vi "Get Stock Prices.vi"(11 "time":i32) -> (3 "Prices":dbl[](array[numeric]))   [LabVIEW 2025, in "Full Featured MCP Server.lvlib"]
doc: "Teturns all prices of the stocks for a specific point in time. Use this twice to compare price changes."
uses:
  Full Featured MCP Server.lvlib
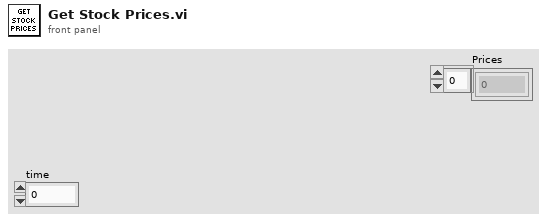
[diagram p1: front panel]
types:
  T1 = typedef "Full Featured MCP Server.lvlib/Server Data.ctl" = cluster{"Stocks Prices":dbl[][], "Owned Stocks":i32[], "Stock Names":string[], "Wallet":dbl, "Fluctuation":dbl, "Stock Trends":dbl[]}
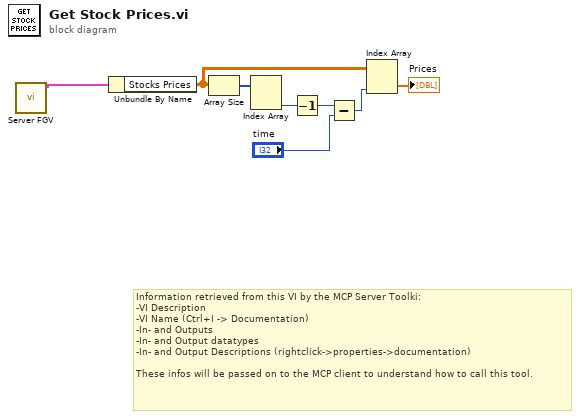
[diagram p0: block diagram]
diagram:
  # "Information retrieved from this VI by the MCP Server Toolki:\n-VI Description\n-VI Name (Ctrl+I -> Documentation)\n-In- and Outputs\n-In- and Output datatypes\n-In- and Output Descriptions (rightclick->properties->documentation)\n\nThese infos will be passed on to the MCP client to understand how to call this tool."
  n1 = call "Server FGV.vi"() -> ("Full Features MCP Server Data"=w1:T1)  [unwired: 9 in, 2 out]
  n2 = Unbundle By Name(w1) -> ("Stocks Prices"=w6:dbl[][])
  n3 = Array Size(array=w6) -> (size(s)=w8:i32[])
  n4 = Index Array(array=w8) -> (element #2=w7:i32)  [unwired: 2 in, 1 out]
  n5 = Decrement(x=w7) -> (x-1=w5:i32)
  n6 = Subtract(x=w5, y="time") -> (x-y=w3:i32)
  n7 = Index Array(array=w6, index (col)=w3) -> (element=→"Prices":dbl[])  [unwired: 1 in]
